vi "ble_read_by_handle.vi"(6 "Connection Status":T1={"MAC Address"="", "cnx handle"=0, "cnx flags"=0, "Address Type"=125, "Connection Interval (ms)"=125, "Timeout(ms)"=125, "Latency"=0, "bonding handle"=0} {"Address Type" items=["Public", "Random"]}, 7 "Handle":u16=1 format="%04x", 8 "error in (no error)":errorcluster, 11 "COM Bluegiga in":refnum<visa-resource-name>) -> (0 "error out":errorcluster, 2 "characteristic value":u8[](array[numeric]), 3 "COM Bluegiga out":refnum<visa-resource-name>)   [LabVIEW 2017]
uses:
  type_def/connection_status_bundle.ctl
  type_def/address_type.ctl
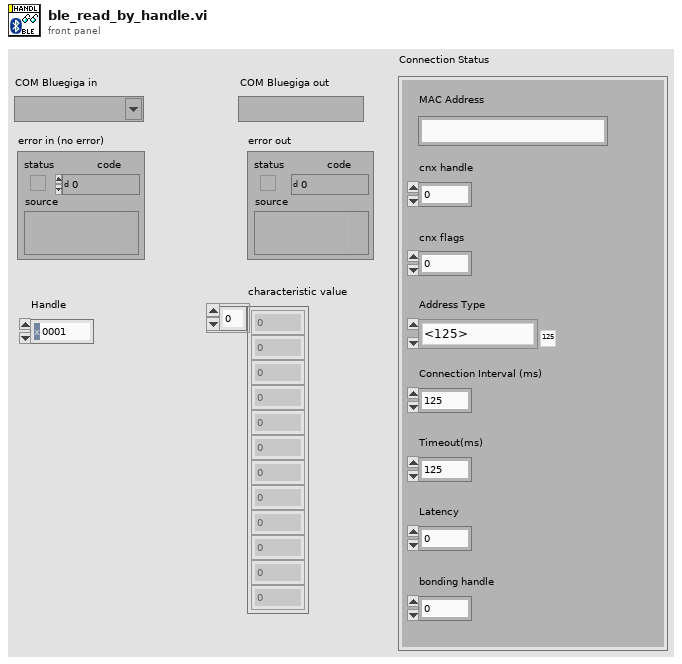
[diagram p1: front panel]
types:
  T1 = typedef "connection_status_bundle.ctl" = cluster{"MAC Address":string, "cnx handle":u8, "cnx flags":u8, "Address Type":T2, "Connection Interval (ms)":u16, "Timeout(ms)":u16, "Latency":u16, "bonding handle":u8}
  T2 = typedef "address_type.ctl" = u8
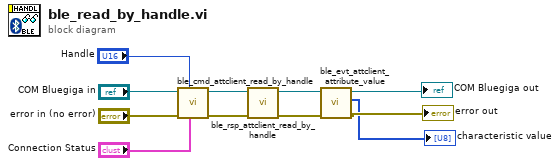
[diagram p0: block diagram]
diagram:
  n1 = call "ble_cmd_attclient_read_by_handle.vi"("Connection Status"="Connection Status", "chrHandle"="Handle", "error in (no error)"="error in (no error)", "COM Bluegiga in"="COM Bluegiga in") -> ("error out"=w8:errorcluster, "COM Bluegiga out"=w9:refnum<visa-resource-name>)  [unwired: 6 in]
  n2 = call "ble_rsp_attclient_read_by_handle.vi"("error in (no error)"=w8, "COM Bluegiga in"=w9) -> ("error out"=w6:errorcluster, "COM Bluegiga out"=w7:refnum<visa-resource-name>)  [unwired: 6 in, 2 out]
  n3 = call "ble_evt_attclient_attribute_value.vi"("error in (no error)"=w6, "COM Bluegiga in"=w7) -> ("error out"=→"error out":errorcluster, "characteristic value"=→"characteristic value":u8[], "COM Bluegiga out"=→"COM Bluegiga out":refnum<visa-resource-name>)  [unwired: 6 in, 1 out]
